vi "基础 2.vi"() -> ()   [LabVIEW 2014]
doc: "计算三个数的平均值"
panel:
  out "平均数":dbl
  in  "C":dbl
  in  "B":dbl
  in  "A":dbl
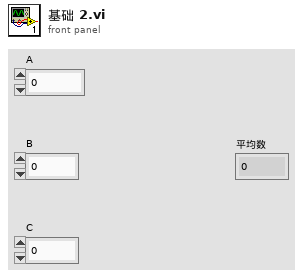
[diagram p1: front panel]
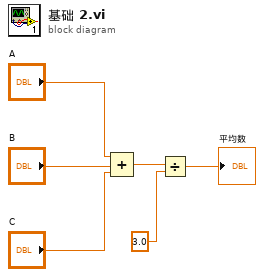
[diagram p0: block diagram]
diagram:
  n1 = Compound Arithmetic op=ADD("A", "B", "C") -> (w2:dbl)
  n2 = Divide(x=w2, y=3.0) -> (x/y=→"平均数":dbl)
